vi "CONFIG NEO ARM ACTUATORS.vi"(8 "error in (no error)":errorcluster, 10 "MotorControlDevRef":T5, 11 "RefName":string) -> (0 "error out":errorcluster)   [LabVIEW 2020]
uses:
  <vilib>/Rock Robotics/WPI/MotorControl/WPI_MotorControlDeviceRef.ctl
  <vilib>/Rock Robotics/WPI/MotorControl/WPI_MotorControlType.ctl
  <vilib>/Rock Robotics/SystemInterfaces/DIO/FPGA_DIOPWMChannel.ctl
  <vilib>/Rock Robotics/WPI/PWM/WPI_PWMDeadband.ctl
  <vilib>/Rock Robotics/SystemInterfaces/DIO/FPGA_DIOChannel.ctl
  <vilib>/Rock Robotics/WPI/ThirdParty/REV Robotics/REVLib/Typedef/Spark MAX Motor Type.ctl
  <vilib>/Rock Robotics/WPI/ThirdParty/REV Robotics/REVLib/Typedef/Spark MAX Sensor Type.ctl
  <vilib>/Rock Robotics/WPI/ThirdParty/REV Robotics/REVLib/Typedef/Spark MAX Idle Mode.ctl
  <vilib>/Rock Robotics/WPI/ThirdParty/REV Robotics/REVLib/Typedef/Spark MAX Limit Switch Polarity.ctl
  <vilib>/Rock Robotics/WPI/ThirdParty/REV Robotics/REVLib/Typedef/Spark MAX Limit Direction.ctl
panel:
  in  "REV Polarity (Normally Open)":T1
  in  "REV Enabled? (T)":bool
  in  "FWD Polarity (Normally Open)":T1
  in  "FWD Enabled? (T)":bool
  out "inches/s per motor rpm":dbl
  out "inches per motor rev":dbl
  in  "Idle Mode":T2=enum."Brake"
  in  "Sensor Type (Hall Sensor)":T3=enum."Hall Sensor"
  in  "Motor Type":T4
  out "gear ratio":dbl
  in  "screw TPI":i32=12
  in  "TEETH - to screw":i32=50
  in  "TEETH - pinion":i32=14
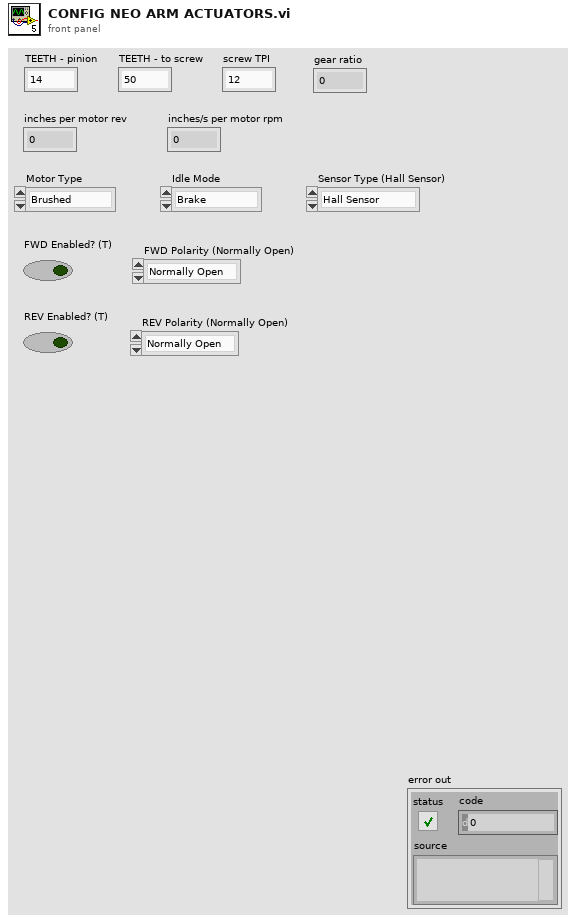
[diagram p1: front panel]
types:
  T1 = typedef "Spark MAX Limit Switch Polarity.ctl" = enum16{"Normally Open", "Normally Closed"}
  T2 = typedef "Spark MAX Idle Mode.ctl" = enum16{"Coast", "Brake"}
  T3 = typedef "Spark MAX Sensor Type.ctl" = enum16{"No Sensor", "Hall Sensor", "Encoder", "-Not Available-", "Analog", "Alternate Encoder"}
  T4 = typedef "Spark MAX Motor Type.ctl" = enum16{"Brushed", "Brushless"}
  T5 = typedef "WPI_MotorControlDeviceRef.ctl" = cluster{"DeviceStatus":errorcluster, "Type":T6, "PWM":cluster{"PWM Channel":T7, "DeadBand":T8}, "CAN":cluster{"Device Number":u8, "SetOutput VI Ref":variant, "GetOutput VI Ref":variant, "Enable VI Ref":variant, "Disable VI Ref":variant, "Data":variant}, "Invert":bool, "DIO PWM":cluster{"PWM \"Enable\" Channel":T7, "DIOChannel":T9, "PWM Rate":dbl}}
  T6 = typedef "WPI_MotorControlType.ctl" = enum16{"PWM", "CAN", "DIO PWM"}
  T7 = typedef "FPGA_DIOPWMChannel.ctl" = enum8{"PWM 0", "PWM 1", "PWM 2", "PWM 3", "PWM 4", "PWM 5", "PWM 6", "PWM 7", "PWM 8", "PWM 9", "PWM MXP 0", "PWM MXP 1", "PWM MXP 2", "PWM MXP 3", "PWM MXP 4", "PWM MXP 5", "PWM MXP 6", "PWM MXP 7", "PWM MXP 8", "PWM MXP 9", "Invalid"}
  T8 = typedef "WPI_PWMDeadband.ctl" = cluster{"Name":string, "maxPositivePwm":i32, "minPositivePwm":i32, "centerPwm":i32, "maxNegativePwm":i32, "minNegativePwm":i32, "angularRange":u16}
  T9 = typedef "FPGA_DIOChannel.ctl" = enum8{"DIO 0", "DIO 1", "DIO 2", "DIO 3", "DIO 4", "DIO 5", "DIO 6", "DIO 7", "DIO 8", "DIO 9", "DIO MXP 0", "DIO MXP 1", "DIO MXP 2", "DIO MXP 3", "DIO MXP 4", "DIO MXP 5", "DIO MXP 6", "DIO MXP 7", "DIO MXP 8", "DIO MXP 9", "DIO MXP 10", "DIO MXP 11", "DIO MXP 12", "DIO MXP 13", "DIO MXP 14", "DIO MXP 15", "SPI Port CS1", "SPI Port CS2", "SPI Port CS3", "SPI Port MISO", "SPI Port MOSI", "Invalid"}
  T10 = typedef "Spark MAX Limit Direction.ctl" = enum16{"Forward Limit", "Reverse Limit"}
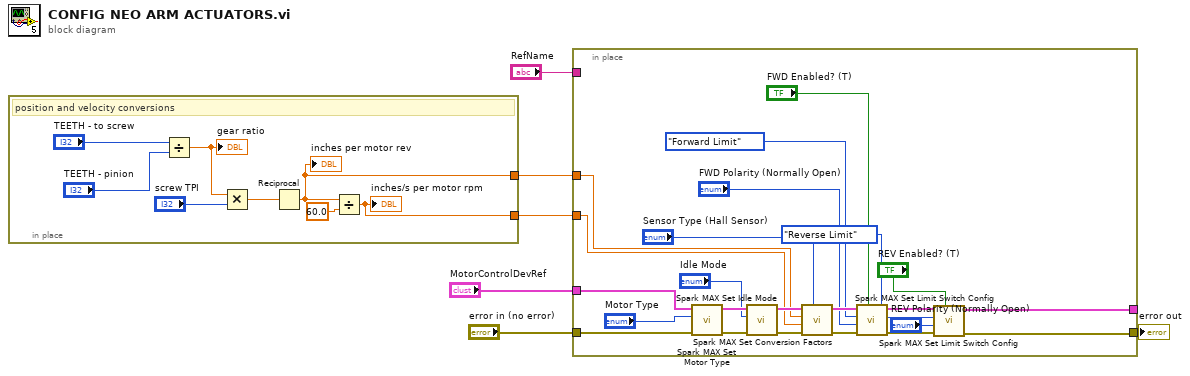
[diagram p0: block diagram]
diagram:
  n1 = in-place {
    in-place-border: [w8] -> w2
    in-place-border: [w7] -> w1
    # "position and velocity conversions"
    n2 = Divide(x="TEETH - to screw", y="TEETH - pinion") -> (x/y=w10:dbl)
    "gear ratio" <- w10
    n3 = Multiply(x=w10, y="screw TPI") -> (x*y=w11:dbl)
    n4 = Reciprocal(x=w11) -> (1/x=w8:dbl)
    "inches per motor rev" <- w8
    n5 = Divide(x=w8, y=60.0) -> (x/y=w7:dbl)
    "inches/s per motor rpm" <- w7
  }
  n6 = in-place {
    in-place-border: "MotorControlDevRef" -> [w37]
    in-place-border: [w19] -> w4
    in-place-border: "error in (no error)" -> [w34]
    in-place-border: "RefName" -> [_]
    in-place-border: w2 -> [w28]
    in-place-border: w1 -> [w27]
    in-place-border: [w18] -> _
    n7 = call <vilib>:"Spark MAX Set Motor Type.vi"("error in (no error)"=w34, "Motor Type"="Motor Type", "MotorControlDevRef"=w37) -> ("error out"=w33:errorcluster, "MotorControlDeviceRef"=w36:T5)  [unwired: 7 in]
    n8 = call <vilib>:"Spark MAX Set Idle Mode.vi"("error in (no error)"=w33, "Idle Mode"="Idle Mode", "MotorControlDeviceRef in"=w36) -> ("error out"=w32:errorcluster, "MotorControlDeviceRef out"=w35:T5)  [unwired: 7 in]
    n9 = call <vilib>:"Spark MAX Set Conversion Factors.vi"("Sensor Type (Hall Sensor)"="Sensor Type (Hall Sensor)", "error in (no error)"=w32, "Velocity Factor (1)"=w27, "Position Factor (1)"=w28, "MotorControlDeviceRef in"=w35) -> ("error out"=w25:errorcluster, "MotorControlDeviceRef out"=w26:T5)  [unwired: 5 in]
    n10 = call <vilib>:"Spark MAX Set Limit Switch Config.vi"("Enabled? (T)"="FWD Enabled? (T)", "error in (no error)"=w25, "Polarity (Normally Open)"="FWD Polarity (Normally Open)", "Limit Switch"=Spark_MAX_Limit_Direction."Forward Limit" ("FWD Limit Switch"), "MotorControlDeviceRef in"=w26) -> ("error out"=w20:errorcluster, "MotorControlDeviceRef out"=w21:T5)  [unwired: 5 in]
    n11 = call <vilib>:"Spark MAX Set Limit Switch Config.vi"("Enabled? (T)"="REV Enabled? (T)", "error in (no error)"=w20, "Polarity (Normally Open)"="REV Polarity (Normally Open)", "Limit Switch"=Spark_MAX_Limit_Direction."Reverse Limit", "MotorControlDeviceRef in"=w21) -> ("error out"=w19:errorcluster, "MotorControlDeviceRef out"=w18:T5)  [unwired: 5 in]
  }
  "error out" <- w4
